vi "PV ActiveLine - FullScaleRange (TPG361).vi"(7 "W/R":bool, 8 "Fehler (Eingang)":errorcluster, 10 "Sensor 1 Set":i8(ring)=3 items=["0.01 mbar", "0.1 mbar", "1 mbar", "10 mbar", "100 mbar", "1000 mbar", "2 bar", "5 bar", "10 bar", "50 bar"], 11 "Referenz in":refnum<visa-resource-name>) -> (0 "Cluster (Ausgang)":errorcluster, 2 "Sensor 1 Get":i8(ring)=3 items=["0.01 mbar", "0.1 mbar", "1 mbar", "10 mbar", "100 mbar", "1000 mbar", "2 bar", "5 bar", "10 bar", "50 bar"], 3 "Referenz out":refnum<visa-resource-name>)   [LabVIEW 2013, in "PV ActiveLine.lvlib"]
doc: "FSR - Measurement Range (F.S.) of Linear Gauges [hPa = mbar]\n\nTransmit: FSR [,a]\nReceive: a\n\nFull scale value gauge 1, a =\n0 –> 0.01 hPa\n1 –> 0.1 hPa\n2 –> 1 hPa\n3 –> 10 hPa\n4 –> 100 hPa\n5 –> 1000 hPa (default)\n6 –> 200 kPa\n7 –> 500 kPa\n8 –> 1000 kPa\n9 –> 5000 kPa\n\nThe full scale value of the measurement range (Full Scale) of linear gauges has to be defined by the user; the full scale value of logarithmic gauges is automatically recognized."
uses:
  C:/Program Files (x86)/National Instruments/LabVIEW 2013/PV ActiveLine/PV ActiveLine.lvlib
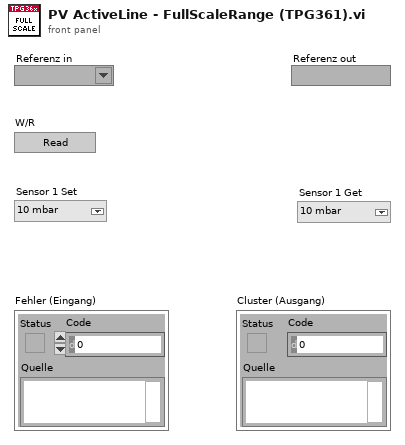
[diagram p1: front panel]
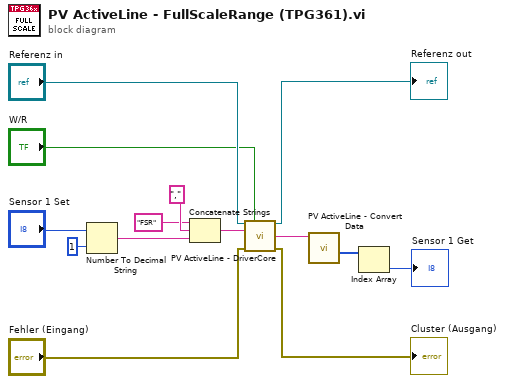
[diagram p0: block diagram]
diagram:
  n1 = Number To Decimal String(number="Sensor 1 Set", width (-)=i16 1) -> (decimal integer string=w9:string)
  n2 = Concatenate Strings("FSR", ",", w9) -> (w6:string)
  n3 = call "PV ActiveLine - DriverCore.vi"("Referenz in"="Referenz in", "Write/Read"="W/R", "Command"=w6, "Fehler (Eingang)"="Fehler (Eingang)") -> ("Referenz out"=→"Referenz out":refnum<visa-resource-name>, "String Out"=w3:string, "Cluster (Ausgang)"=→"Cluster (Ausgang)":errorcluster)  [unwired: 9 in]
  n4 = call "PV ActiveLine - Convert Data.vi"("String in"=w3) -> ("Integer Out"=w2:i32[])  [unwired: 7 in, 3 out]
  n5 = Index Array(array=w2) -> (element=→"Sensor 1 Get":i32)  [unwired: 1 in]
